vi "Configure Modulation (Amplitude).vi"(0 "VISA resource name":refnum<visa-resource-name>, 1 "Enable Amplitude Modulation (T:Enable)":bool, 2 "Modulation Frequency (1000.0 Hz)":dbl, 5 "Channel (1: Channel1)":u16(ring) items=["Channel1", "Channel2"], 7 "AM Source (0: Internal)":u16(ring) items=["Internal", "Other Channel", "External"], 9 "Modulation Waveform (0: Sine)":u16(ring) items=["Sine", "Square", "Ramp", "Negative Ramp", "Triangle", "Noise", "Arbitrary Waveform"], 11 "error in (no error)":errorcluster, 12 "Arbitrary Waveform Name (\"ARB1\")":string, 13 "Modulation Depth (100.0 %)":dbl, 14 "Enable Carrier Suppression (F: Disable)":bool) -> (4 "VISA resource name out":refnum<visa-resource-name>, 15 "error out":errorcluster)   [LabVIEW 2009, in "Agilent 81150.lvlib"]
doc: "Configures and enables amplitude modulation (AM). In AM, the amplitude of the carrier is varied by the amplitude of the modulating waveform. \n\n<B>Note(s):</B>\nThe carrier waveform shape and parameters are set by the Configure Standard Waveform VI."
uses:
  Agilent 81150.lvlib
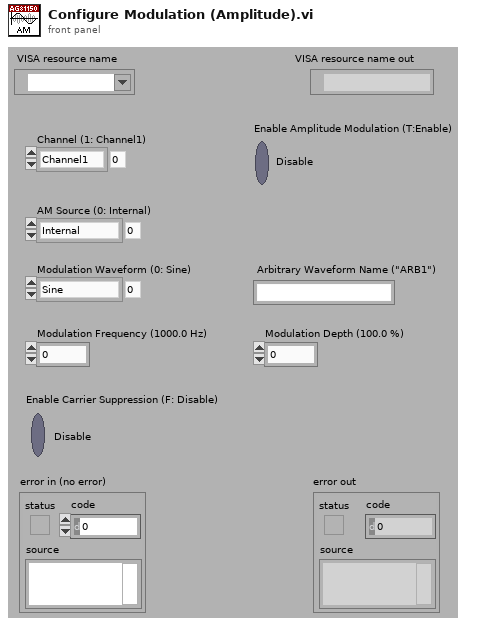
[diagram p1: front panel]
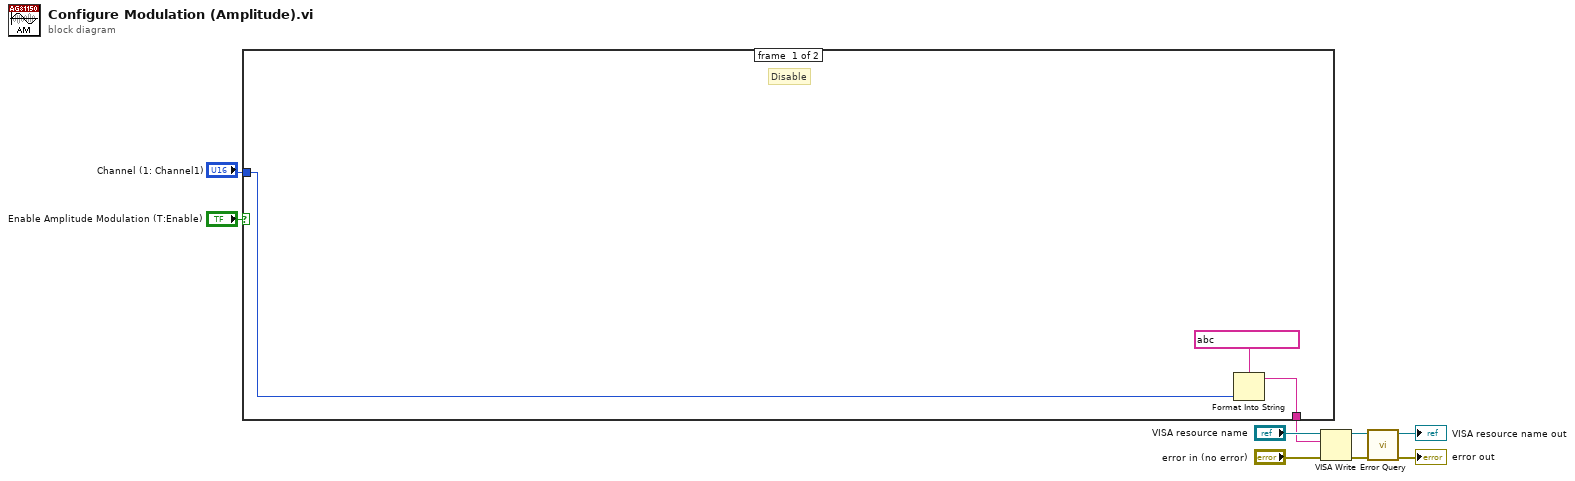
[diagram p0: block diagram]
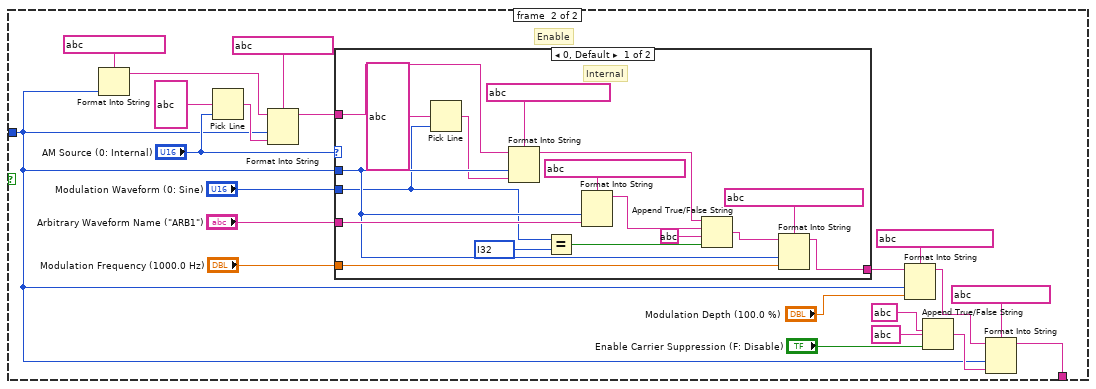
[diagram p2: hidden frame]
diagram:
  n1 = case shown="True" "Enable Amplitude Modulation (T:Enable)" {
    tunnel: [w11 w13] -> w3
    tunnel: "Channel (1: Channel1)" -> [w10 w15]
    frame #0 {
      # "Disable"
      n2 = Format Into String(format string=string ?, w10) -> (resulting string=w11:string)  [unwired: 2 in, 1 out]
    }
    frame #1 {
      # "Enable"
      n3 = Format Into String(format string=string ?, w15) -> (resulting string=w14:string)  [unwired: 2 in, 1 out]
      n4 = Pick Line(multi-line string=string ?, line index="AM Source (0: Internal)") -> (output string=w17:string)  [unwired: 1 out]
      n5 = Format Into String(format string=string ?, initial string=w14, w15, w17) -> (resulting string=w19:string)  [unwired: 1 in, 1 out]
      n6 = case shown="0, Default" "AM Source (0: Internal)" {
        tunnel: w15 -> [w44 _]
        tunnel: [w47 w51] -> w32
        tunnel: "Modulation Waveform (0: Sine)" -> [w35 _]
        tunnel: "Modulation Frequency (1000.0 Hz)" -> [w46 _]
        tunnel: "Arbitrary Waveform Name (\"ARB1\")" -> [w45 _]
        tunnel: w19 -> [w36 w51]
        frame #0 {
          w34 = i32 ? items=["Sine", "Square", "Ramp", "Negative Ramp", "Triangle", "Noise", "User"] ("Modulation Waveform (0: Sine) 2")
          # "Internal"
          n7 = Pick Line(multi-line string=string ?, line index=w35) -> (output string=w42:string)  [unwired: 1 out]
          n8 = Format Into String(format string=string ?, initial string=w36, w44, w42) -> (resulting string=w40:string)  [unwired: 1 in, 1 out]
          n9 = Equal?(x=w35, y=w34) -> (x = y?=w41:bool)
          n10 = Format Into String(format string=string ?, w44, w45) -> (resulting string=w39:string)  [unwired: 2 in, 1 out]
          n11 = Append True/False String(1:w41, 2:string ?, 3:w39, 4:w40) -> (0:w38:string)
          n12 = Format Into String(format string=string ?, initial string=w38, w44, w46) -> (resulting string=w47:string)  [unwired: 1 in, 1 out]
        }
        frame #1 {
          # "Other Channel or External"
        }
      }
      n13 = Format Into String(format string=string ?, initial string=w32, w15, "Modulation Depth (100.0 %)") -> (resulting string=w28:string)  [unwired: 1 in, 1 out]
      n14 = Append True/False String(1:"Enable Carrier Suppression (F: Disable)", 2:string ?, 3:string ?) -> (0:w23:string)  [unwired: 1 out]
      n15 = Format Into String(format string=string ?, initial string=w28, w15, w23) -> (resulting string=w13:string)  [unwired: 1 in, 1 out]
    }
  }
  n16 = VISA Write(VISA resource name="VISA resource name", write buffer=w3, error in (no error)="error in (no error)") -> (VISA resource name out=w5:refnum<visa-resource-name>, error out=w4:errorcluster)  [unwired: 1 out]
  n17 = call "Error Query.vi"("error in (no error)"=w4, "VISA resource name"=w5) -> ("error out"=→"error out":errorcluster, "VISA resource name out"=→"VISA resource name out":refnum<visa-resource-name>)  [unwired: 8 out]
